vi "GetMenuDisplayed.vi"(8 "error in (no error)":errorcluster, 10 "Tag":string, 11 "Menu in":refnum<class "Menu.lvclass">) -> (0 "error out":errorcluster, 2 "Displayed?":bool, 3 "Menu out":refnum<class "Menu.lvclass">)   [LabVIEW 2021, in "Menu.lvlib" / "Menu.lvclass"]
uses:
  Menu.lvclass
  <vilib>/Utility/error.llb/Error Cluster From Error Code.vi
  <vilib>/ErrorRing/Error Ring.xnode
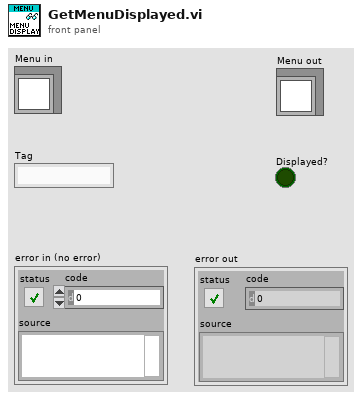
[diagram p1: front panel]
types:
  T1 = typedef "Menu.lvlib/Menu.lvclass/Data.ctl" = cluster{"MenuMap":map{string, T2}, "PictRef":refnum<vi>, "MenuSelectionEvent":refnum<user-event>, "TopMenuSpacing":i32, "MenuSpacing":i32, "CloseEvent":refnum<user-event>, "TR_ManageMenuRef":refnum<vi>, "MenuColors":T4, "RTMPath":path, "RTMVIReference":refnum<vi>, "RTMMenuReference":refnum<k9>, "CtlRef":refnum<vi>, "User-Specified Font":refnum<class "Font.lvclass">, "Desired Font":enum16{"User-specified Font", "Application Font", "System Font", "Dialog Font"}, "SubMenuIcon":T5, "SubMenuIconClosed":refnum<class "Picture2D.lvclass">, "SubMenuIconOpened":refnum<class "Picture2D.lvclass">}
  T2 = typedef "Menu.lvlib/Menu.lvclass/MenuItems.ctl" = cluster{"Item Name":string, "Short Cut":T3, "Checked":bool, "Enable":bool, "After item":string, "Item Tags":string[], "Item Names":string[], "Picture":refnum<class "Image.lvclass">, "Hilite Picture":refnum<class "Image.lvclass">, "Displayed":bool}
  T3 = typedef "LVMenuShortCut.ctl" = cluster{"Include Shift Key?":bool, "Include Ctrl Key?":bool, "Shortcut Key":string}
  T4 = typedef "Menu.lvlib/Menu.lvclass/MenuColors.ctl" = cluster{"Text":refnum<class "Color.lvclass">, "HiliteText":refnum<class "Color.lvclass">, "Background":refnum<class "Color.lvclass">, "BorderColor":refnum<class "Color.lvclass">, "Hilite":refnum<class "Color.lvclass">}
  T5 = typedef "Menu.lvlib/Menu.lvclass/SubMenuIcon.ctl" = enum16{"LabVIEW", "Windows", "Custom"}
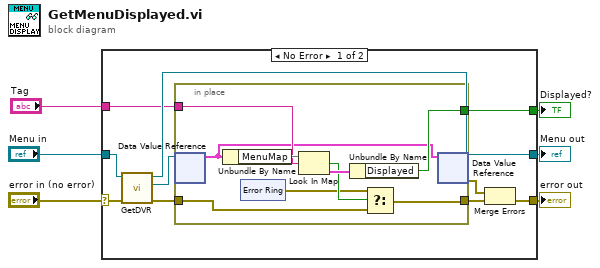
[diagram p0: block diagram]
diagram:
  n1 = case shown="No Error" "error in (no error)" {
    selector: "error in (no error)" -> [w11 w30]
    tunnel: "Menu in" -> [w16 w31]
    tunnel: [w9 w31] -> w4
    tunnel: [w10 w30] -> w3
    tunnel: [w8 _] -> w2
    tunnel: "Tag" -> [w7 _]
    frame No Error {
      n2 = call "GetDVR.vi"("error in (no error)"=w11, "Menu in"=w16) -> ("error out"=w15:errorcluster, "DVR"=w14:refnum<data-value>, "Menu out"=w9:refnum<class "Menu.lvclass">)  [unwired: 7 in]
      n3 = in-place {
        in-place-border: w15 -> [w17]
        in-place-border: [w20] -> w13
        in-place-border: [w23] -> w8
        in-place-border: w7 -> [w22]
        n4 = in-place-dvr #1(w14) -> (w21:T1)  [unwired: 1 out]
        n5 = Unbundle By Name(w21) -> ("MenuMap"=w25:map{string, T2})
        n6 = xnode "Error Ring"() -> ("error out"=w18:errorcluster)
        n7 = Look In Map(map=w25, key=w22) -> (key not found?=w19:bool, value=w24:T2)  [unwired: 1 in]
        n8 = Unbundle By Name(w24) -> ("Displayed"=w23:bool)
        n9 = Select(t=w18, s=w19, f=w17) -> (s? t:f=w20:errorcluster)
        n10 = in-place-dvr #1(w21) -> (w12:errorcluster)  [unwired: 1 out]
      }
      n11 = Merge Errors(w12, w13) -> (w10:errorcluster)
    }
    frame Error {
    }
  }
  "Menu out" <- w4
  "error out" <- w3
  "Displayed?" <- w2
